vi "LVProjectShortcut_Item_OnPopupMenu.vi"(11 "Object":T1) -> ()   [LabVIEW 2017, in "LVProject Shortcut.lvlib"]
uses:
  <resource>/Framework/Providers/API/ItemRef.ctl
  <resource>/Framework/Providers/API/mxLvMenuItem.ctl
  LVProject Shortcut.lvlib
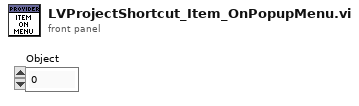
[diagram p1: front panel]
types:
  T1 = typedef "ItemRef.ctl" = u64
  T2 = typedef "mxLvMenuItem.ctl" = cluster{"Menu Name":string, "Description":string, "Icon File Name":path, "Menu Tag":string, "Enabled":bool, "Checked":bool, "Separator":bool, "Batchable":bool, "Weight":i32, "Batch Mode (Ignored if Not Batchable)":enum32{"Show If All Items Support Command", "Show If Any Items Support Command"}, "Menu Location":enum32{"<None>", "Project", "Project / Build Specifications", "Tools", "Tools / Source Control", "Tools / Real-Time Module", "Help"}, "Exclude From Getting Started Window Menu":bool}
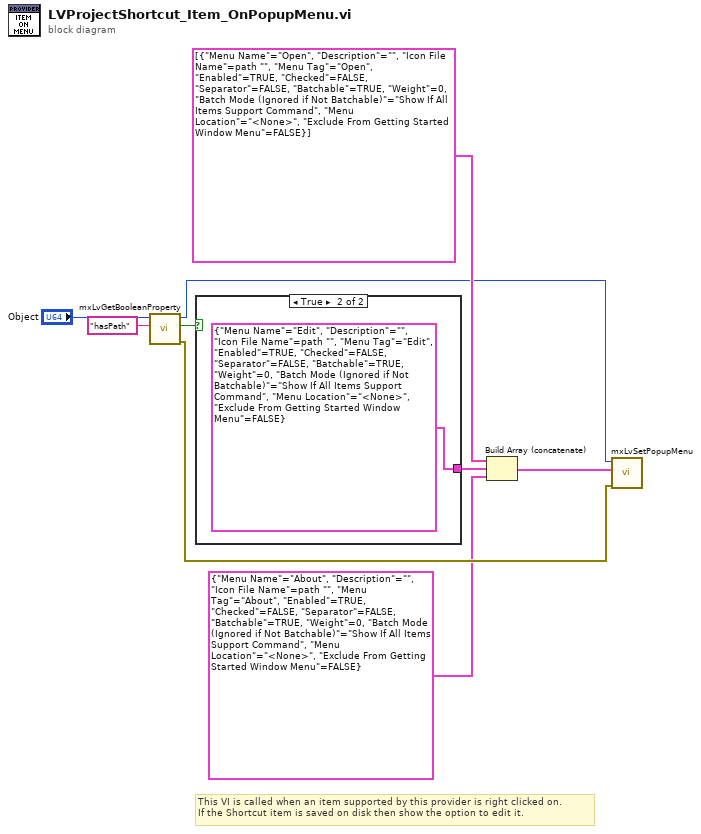
[diagram p0: block diagram]
diagram:
  # "This VI is called when an item supported by this provider is right clicked on.\nIf the Shortcut item is saved on disk then show the option to edit it."
  n1 = call <resource>:"mxLvGetBooleanProperty.vi"("Tag"="hasPath", "Item"="Object") -> ("error out"=w6:errorcluster, "Value"=w1:bool, "Item"=w7:T1)  [unwired: 7 in]
  n2 = case shown="True" w1 {
    tunnel: [_ T2 {"Menu Name"="Edit", "Description"="", "Icon File Name"=path "", "Menu Tag"="Edit", "Enabled"=TRUE, "Checked"=FALSE, "Separator"=FALSE, "Batchable"=TRUE, "Weight"=0, "Batch Mode (Ignored if Not Batchable)"=enum."Show If All Items Support Command", "Menu Location"=enum."<None>", "Exclude From Getting Started Window Menu"=FALSE} ("Menu Item")] -> w2
    frame False {
    }
    frame True {
    }
  }
  n3 = Build Array (concatenate)(T2[] [{"Menu Name"="Open", "Description"="", "Icon File Name"=path "", "Menu Tag"="Open", "Enabled"=TRUE, "Checked"=FALSE, "Separator"=FALSE, "Batchable"=TRUE, "Weight"=0, "Batch Mode (Ignored if Not Batchable)"=enum."Show If All Items Support Command", "Menu Location"=enum."<None>", "Exclude From Getting Started Window Menu"=FALSE}] ("Popup Menu Items"), w2, T2 {"Menu Name"="About", "Description"="", "Icon File Name"=path "", "Menu Tag"="About", "Enabled"=TRUE, "Checked"=FALSE, "Separator"=FALSE, "Batchable"=TRUE, "Weight"=0, "Batch Mode (Ignored if Not Batchable)"=enum."Show If All Items Support Command", "Menu Location"=enum."<None>", "Exclude From Getting Started Window Menu"=FALSE} ("Menu Item")) -> (w8:T2[])
  n4 = call <resource>:"mxLvSetPopupMenu.vi"("error in"=w6, "Popup Menu Items"=w8, "Item"=w7) -> ()  [unwired: 7 in, 2 out]
